vi "getDeviceType.vi"(8 "error in (no error)":errorcluster, 11 "AnalogDevice.lvclass in":refnum<class "AnalogDevice.lvclass">) -> (0 "error out":errorcluster, 2 "type":T1(ring), 3 "AnalogDevice.lvclass out":refnum<class "AnalogDevice.lvclass">)   [LabVIEW 2011, in "Tools.lvlib" / "DatabaseHelpers.lvlib" / "AnalogDevice.lvclass"]
uses:
  AnalogDevice.lvclass
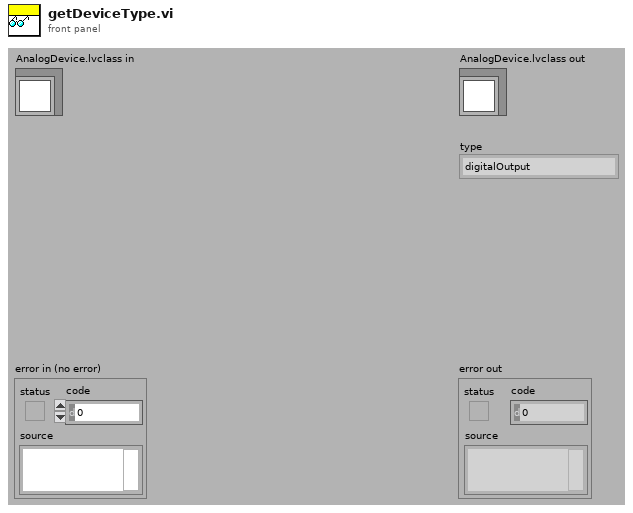
[diagram p1: front panel]
types:
  T1 = enum16{"digitalOutput", "digitalInput", "analogOutput", "analogInput", "rfOutput", "ethernetSupply"}
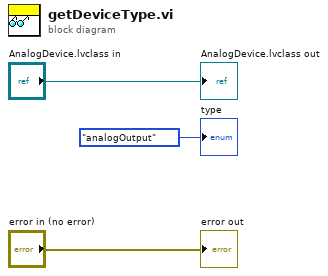
[diagram p0: block diagram]
diagram:
  "error out" <- "error in (no error)"
  "AnalogDevice.lvclass out" <- "AnalogDevice.lvclass in"
  "type" <- T1."analogOutput" ("type")
